vi "Open DataTable.vi"(6 "visible (false)":bool=TRUE, 8 "error in (no error)":errorcluster, 10 "DataTable path":path, 11 "JMP application":refnum<k7>) -> (0 "error out":errorcluster, 2 "DataTable":refnum<k7>, 3 "JMP application out":refnum<k7>)   [LabVIEW 2019, in "JMP Automation.lvlib"]
doc: "Open a new DataTable\n\nJMP application: valide JMP application handle\nvisible (false): if true the table will be visible\nDataTable path: path to the JMP data table file"
uses:
  JMP Automation.lvlib
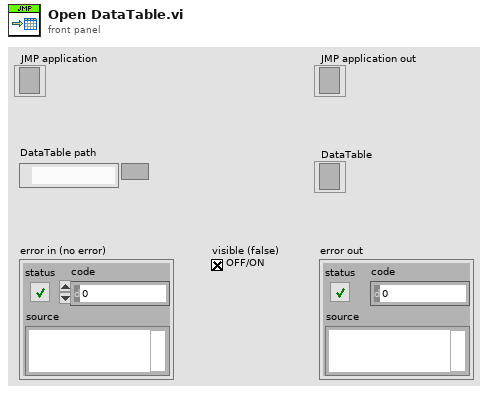
[diagram p1: front panel]
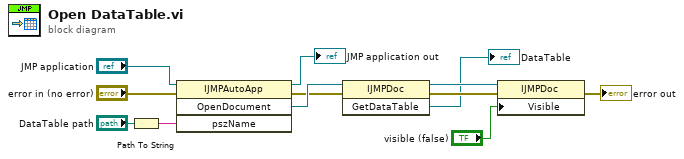
[diagram p0: block diagram]
diagram:
  n1 = Path To String(path="DataTable path") -> (string=w7:string)
  n2 = invoke class="IJMPAutoApp" method="OpenDocument"(reference="JMP application", error in="error in (no error)", "pszName"=w7) -> (reference out=→"JMP application out":refnum<k7>, error out=w2:errorcluster, "OpenDocument"=w5:refnum<k7>)  [unwired: 1 in, 1 out]
  n3 = invoke class="IJMPDoc" method="GetDataTable"(reference=w5, error in=w2) -> (reference out=w4:refnum<k7>, error out=w3:errorcluster, "GetDataTable"=→"DataTable":refnum<k7>)  [unwired: 1 in]
  n4 = property class="IJMPDoc"(reference=w4, error in=w3, "Visible"="visible (false)") -> (error out=→"error out":errorcluster)  [unwired: 1 out]
